vi "SetTask.vi"(8 "error in (no error)":errorcluster, 10 "task":refnum<k21>, 11 "Subsystem":refnum<class "DAQmx(AI).lvclass">) -> (0 "error out":errorcluster, 3 "Subsystem out":refnum<class "DAQmx(AI).lvclass">)   [LabVIEW 2019, in "DAQmx(AI).lvclass"]
doc: "---------------------------------------------------------------\nJKI State Machine Objects™\nhttp://jki.net/state-machine-objects/\nCopyright (C) 2005-2015, JKI <info@jki.net>\nALL RIGHTS RESERVEDJKI State Machine Objects (SMO) 1.0.0.5\nJKI - JKI\nCopyright (c) 2016, JKI"
uses:
  DAQmx(AI).lvclass
  DAQmx(AI).lvclass/DAQmx(AI).ctl
panel:
  # "For instructions on how to use the JKI State Machine Objects, examples and video tutorials, visit:\nhttp://jki.net/state-machine-objects/\n\nJKI State Machine Objects™\nhttp://jki.net/state-machine-objects/\nCopyright (C) 2005-2015, JKI <info@jki.net>\nALL RIGHTS RESERVED"
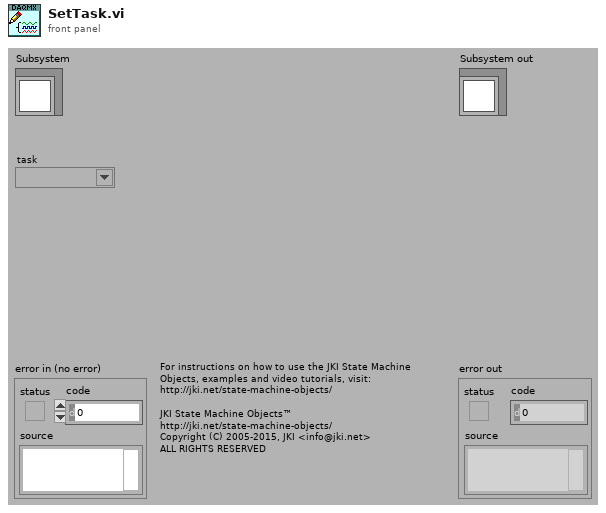
[diagram p1: front panel]
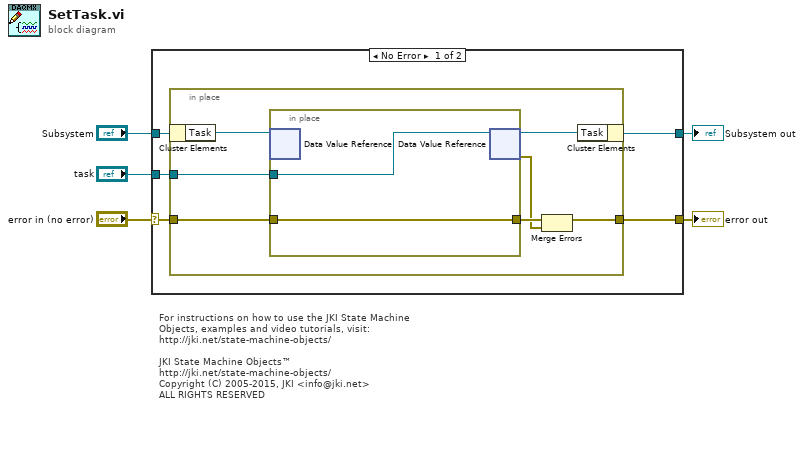
[diagram p0: block diagram]
diagram:
  # "For instructions on how to use the JKI State Machine Objects, examples and video tutorials, visit:\nhttp://jki.net/state-machine-objects/\n\nJKI State Machine Objects™\nhttp://jki.net/state-machine-objects/\nCopyright (C) 2005-2015, JKI <info@jki.net>\nALL RIGHTS RESERVED"
  n1 = case shown="No Error" "error in (no error)" {
    selector: "error in (no error)" -> [w9 w20]
    tunnel: "Subsystem" -> [w10 w21]
    tunnel: [w6 w20] -> w4
    tunnel: [w8 w21] -> w3
    tunnel: "task" -> [w7 _]
    frame No Error {
      n2 = in-place {
        in-place-border: w9 -> [w17]
        in-place-border: [w15] -> w6
        in-place-border: w7 -> [w12]
        n3 = in-place-cluster #1(w10) -> ("Task"=w14:refnum<data-value>)
        n4 = in-place {
          in-place-border: w17 -> [w19]
          in-place-border: [w19] -> w16
          in-place-border: w12 -> [w18]
          n5 = in-place-dvr #2(w14) -> ()  [unwired: 2 out]
          n6 = in-place-dvr #2(w18) -> (w13:refnum<data-value>, w11:errorcluster)
        }
        n7 = Merge Errors(w16, w11) -> (w15:errorcluster)
        n8 = in-place-cluster #1("Task"=w13) -> (w8:refnum<class "DAQmx(AI).lvclass">)
      }
    }
    frame Error {
    }
  }
  "error out" <- w4
  "Subsystem out" <- w3
